vi "TEST low-pass filter.vi"() -> ()   [LabVIEW 2023]
panel:
  out "Hz":dbl=13.333333333333334
  in  "delay between\nchanges (ms)":dbl=75.0 format="%#_13g"
  out "time (s)":dbl=0.2
  out "MAX dx":dbl=2.0
  in  "min value":dbl=-1.0 format="%#_13g"
  in  "max value":dbl=1.0 format="%#_13g"
  out "XY Graph":cluster{dbl[], dbl[]}[](graph)=[{[5.22021999153488, 51.52278871604786, 73.38157823702605, 91.77342481405267, 150.78167335185705, 174.40421511717352, 239.74890369113479, 247.98436852450612, 259.7349960809192, 288.0181687866351, 362.3207131412321, 430.85704379498634, 467.0542828455753, 486.1150660570154, 514.8148552759599, 580.9243575106921, 595.6776684190439, 600.4574203820841, 618.0844251509956, 691.0103653694764, 726.9106386041483, 763.347710475593, 804.9269017654151, 829.4176154781135, 900.1755228714851, 919.2104725342227, 932.1793283342481, 968.6311926677936, 999.1807803129655, 1013.4305338634135, 1057.368996040607, 1066.1285055082517, 1102.7201369970596, 1115.9620241622988, 1190.671281002262, 1232.803430381905, 1291.6692293128892, 1345.9862898242723, 1417.2086982514525, 1452.4089206651893, 1488.2503054329156, 1532.002351889694, 1568.9251703903838, 1625.8058026895037, 1669.4514040612519, 1696.2345529721536, 1743.2673038515697, 1777.3625381699098, 1852.1255644319879, 1889.120280015488], [0.8782582359020026, -0.9188079281250454, 0.1445631652016619, 0.1398141819882941, -0.038244813721349136, -0.7907269009477997, -0.22884217437061327, -0.8492298051288714, 0.7045150718628144, -0.47234266180514206, -0.7777560217891937, -0.6059433608898948, -0.7379329287527652, 0.7847246923994216, 0.4739593404371112, -0.6394059941051622, 0.1744480039916514, -0.8749998854424232, 0.6504870377865277, -0.5623204193652125, -0.9215113780453112, 0.34490476740834675, -0.8323922677529323, -0.5039216337427606, 0.23594614151311966, -0.580529594533298, 0.19531303651227017, -0.4419093615465117, 0.8564583255603875, -0.46878259307810843, 0.7931879234198718, -0.6618303282311624, 0.7333291144717058, 0.6225051125148555, 0.1341740902972175, 0.34335140192232494, 0.5824989130856215, -0.8312873204507425, 0.32361861149384286, 0.06805690914812557, 0.587610398984971, -0.6418359372007543, -0.3532385505641118, -0.5799525009773809, -0.08294167625367521, -0.8381517641336584, 0.13488238098090677, -0.15522065168872246, -0.12715758168076796, 0.3343678086558195]}, {[5.22021999153488, 51.52278871604786, 73.38157823702605, 91.77342481405267, 150.78167335185705, 174.40421511717352, 239.74890369113479, 247.98436852450612, 259.7349960809192, 288.0181687866351, 362.3207131412321, 430.85704379498634, 467.0542828455753, 486.1150660570154, 514.8148552759599, 580.9243575106921, 595.6776684190439, 600.4574203820841, 618.0844251509956, 691.0103653694764, 726.9106386041483, 763.347710475593, 804.9269017654151, 829.4176154781135, 900.1755228714851, 919.2104725342227, 932.1793283342481, 968.6311926677936, 999.1807803129655, 1013.4305338634135, 1057.368996040607, 1066.1285055082517, 1102.7201369970596, 1115.9620241622988, 1190.671281002262, 1232.803430381905, 1291.6692293128892, 1345.9862898242723, 1417.2086982514525, 1452.4089206651893, 1488.2503054329156, 1532.002351889694, 1568.9251703903838, 1625.8058026895037, 1669.4514040612519, 1696.2345529721536, 1743.2673038515697, 1777.3625381699098, 1852.1255644319879, 1889.120280015488], [0.01, -0.04, 0.1445631652016619, 0.1398141819882941, -0.038244813721349136, -0.6282448137213491, -0.3882448137213491, -0.8492298051288714, -0.7592298051288714, -0.6392298051288714, -0.7777560217891937, -0.6059433608898948, -0.7379329287527652, -0.3779329287527652, -0.18793292875276518, -0.48793292875276517, 0.17206707124723486, 0.012067071247234856, 0.06206707124723486, -0.11793292875276513, -0.8579329287527652, -0.4979329287527652, -0.8323922677529323, -0.5039216337427606, -0.26392163374276056, -0.580529594533298, -0.390529594533298, -0.4419093615465117, -0.08190936154651174, -0.39190936154651174, -0.2519093615465117, -0.6618303282311624, -0.5718303282311624, -0.20183032823116243, -0.07183032823116242, 0.34335140192232494, 0.5824989130856215, -0.02750108691437847, 0.32361861149384286, 0.06805690914812557, 0.4180569091481256, 0.05805690914812561, -0.3532385505641118, -0.5799525009773809, -0.08294167625367521, -0.5329416762536752, -0.26294167625367515, -0.15522065168872246, -0.12715758168076796, 0.3343678086558195]}]
  in  "Reset":bool
  in  "Max dx/dt":dbl=10.0
  in  "iterations":i32=50
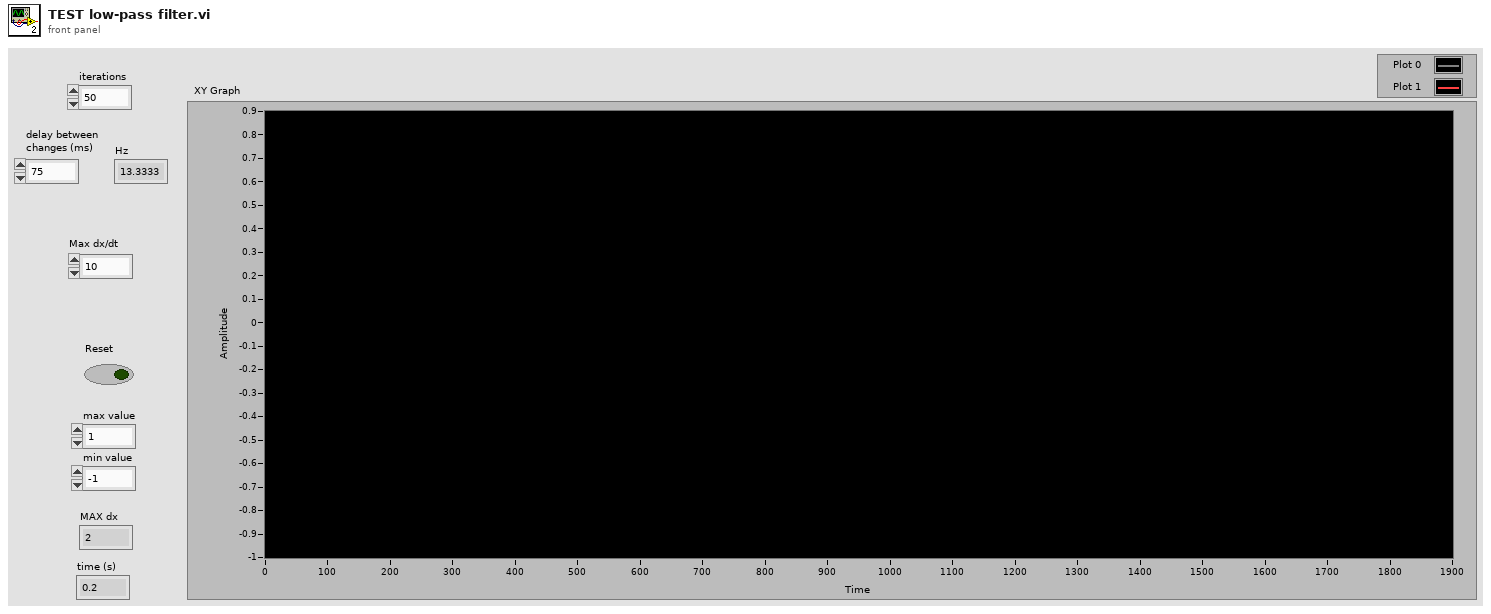
[diagram p1: front panel]
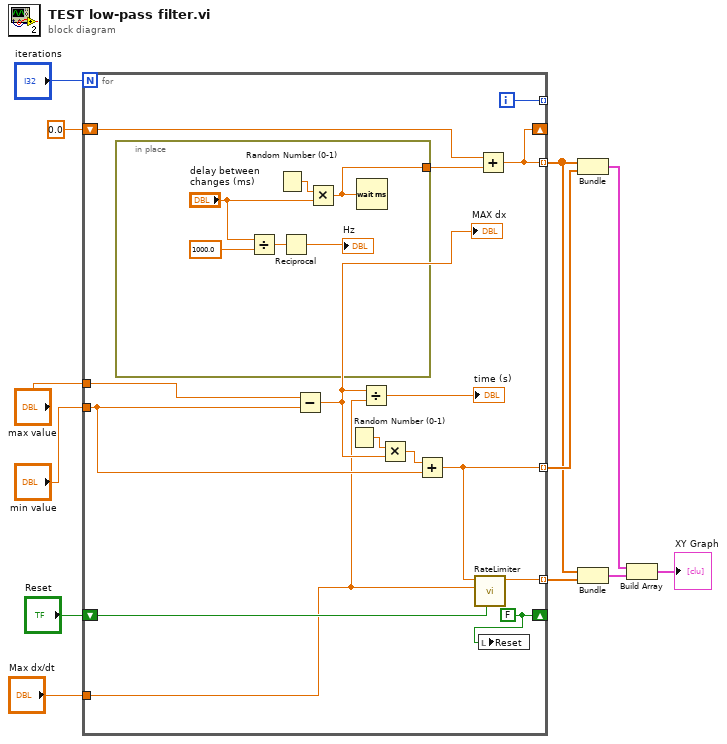
[diagram p0: block diagram]
diagram:
  n1 = for {
    N: "iterations" -> [_]
    tunnel: [w15] -> w11 mode=indexing
    tunnel: [w14] -> w10 mode=indexing
    tunnel: [w25] -> _ mode=indexing
    shift-right: [w22] -> _
    shift-left: 0.0 -> [w24]
    tunnel: [w22] -> w5 mode=indexing
    shift-right: [w13] -> _
    shift-left: "Reset" -> [w19]
    tunnel: "min value" -> [w18]
    tunnel: "max value" -> [w17]
    tunnel: "Max dx/dt" -> [w16]
    i -> [w25]
    w13 = FALSE ("Reset")
    n2 = in-place {
      in-place-border: [w32] -> w23
      n3 = Divide(x="delay between\nchanges (ms)", y=1000.0) -> (x/y=w29:dbl)
      n4 = Random Number (0-1)() -> (number: 0 to 1=w33:dbl)
      n5 = Reciprocal(x=w29) -> (1/x=→"Hz":dbl)
      n6 = Multiply(x=w33, y="delay between\nchanges (ms)") -> (x*y=w32:dbl)
      n7 = Wait (ms)(milliseconds to wait=w32) -> ()  [unwired: 1 out]
    }
    n8 = Subtract(x=w17, y=w18) -> (x-y=w21:dbl)
    "MAX dx" <- w21
    n9 = Random Number (0-1)() -> (number: 0 to 1=w27:dbl)
    n10 = Divide(x=w21, y=w16) -> (x/y=→"time (s)":dbl)
    n11 = Multiply(x=w27, y=w21) -> (x*y=w26:dbl)
    n12 = Add(x=w26, y=w18) -> (x+y=w15:dbl)
    n13 = call "RateLimiter.vi"("Reset"=w19, "Max dx/dt"=w16, "Input"=w15) -> ("Output"=w14:dbl)  [unwired: 8 in]
    n14 = Add(x=w24, y=w23) -> (x+y=w22:dbl)
    n15 = local write "Reset"(w13) -> ()
  }
  n16 = Bundle(w5, w11) -> (w9:cluster{dbl[], dbl[]})  [unwired: 1 in]
  n17 = Bundle(w5, w10) -> (w8:cluster{dbl[], dbl[]})  [unwired: 1 in]
  n18 = Build Array(w9, w8) -> (→"XY Graph":cluster{dbl[], dbl[]}[])
